vi "Free Host.vi"(8 "error in (no error)":errorcluster, 11 "Host":T1) -> (0 "error out":errorcluster)   [LabVIEW 2013, in "libssh2.lvlib"]
uses:
  libssh2.lvlib
  Host Refnum.ctl
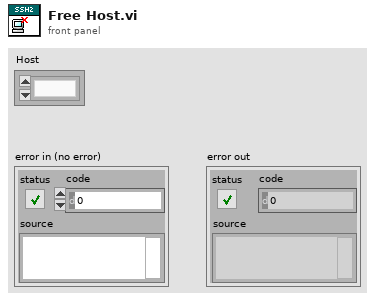
[diagram p1: front panel]
types:
  T1 = typedef "libssh2.lvlib/Host Refnum.ctl" = refnum<k1>
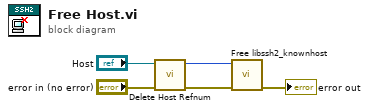
[diagram p0: block diagram]
diagram:
  n1 = call "Delete Host Refnum.vi"("error in (no error)"="error in (no error)", "Host"="Host") -> ("error out"=w5:errorcluster, "libssh2_knownhost*"=w4:u64)  [unwired: 8 in]
  n2 = call "Free libssh2_knownhost.vi"("error in (no error)"=w5, "libssh2_knownhost*"=w4) -> ("error out"=→"error out":errorcluster)  [unwired: 9 in]
